vi "新建模板1.vi"() -> ()   [LabVIEW 2015]
uses:
  <vilib>/vision/NI_Vision_Development_Module.lvlib
  <vilib>/vision/driver/NI_Vision_Acquisition_Software.lvlib
  <vilib>/userdefined/High Color/IMAQdx.ctl
  <vilib>/vision/driver/IMAQdx.llb/IMAQdx Acquisition Mode.ctl
  <vilib>/vision/driver/IMAQdx.llb/IMAQdx Buffer Number Mode.ctl
panel:
  in  "选项卡控件":enum32{"选项卡 1"}(tab)
  out "Image":T1(plugin-control)
  out "Extracted Image":T1(plugin-control)
  in  "Stop":bool
  in  "保存按钮":bool
  in  "布尔":bool
  # "自定义模板界面"
  # "原始图片"
  # "模板图片"
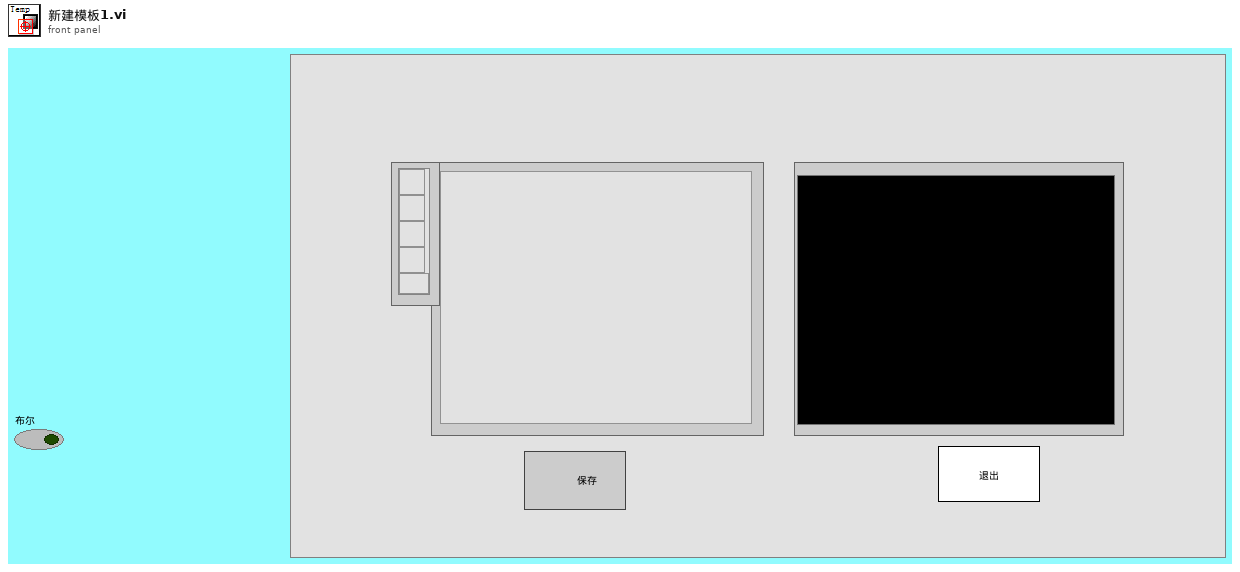
[diagram p1: front panel]
types:
  T1 = typedef "IMAQ Image.ctl" = refnum<image>
  T2 = cluster{"Zoom Tool":bool, "Selection Tool":bool, "Pan Tool":bool, "Point Tool":bool, "Line Tool":bool, "Rectangle Tool":bool, "Rotated Rectangle Tool":bool, "Polyline Tool":bool, "Polygon Tool":bool, "Freehand Tool":bool, "Closed Freehand Tool":bool, "Ellipse Tool":bool, "Annulus Tool":bool}
  T3 = typedef "NI_Vision_Acquisition_Software.lvlib/IMAQdx Buffer Number Mode.ctl" = enum32{"Next", "Last", "Buffer Number", "Every", "Last New"}
  T4 = typedef "NI_Vision_Acquisition_Software.lvlib/IMAQdx Acquisition Mode.ctl" = enum32{"One Shot", "Continuous"}
  T5 = typedef "IMAQdx.ctl" = refnum<k21>
  T6 = cluster{"Match Mode":u16, "Number of Matches Requested":i32, "Minimum Match Score":sgl, "SubPixel Accuracy":bool, "Rotation Angle Ranges":cluster{"Start":sgl, "End":sgl}[], "Show Search Area":bool, "Show Result":bool}
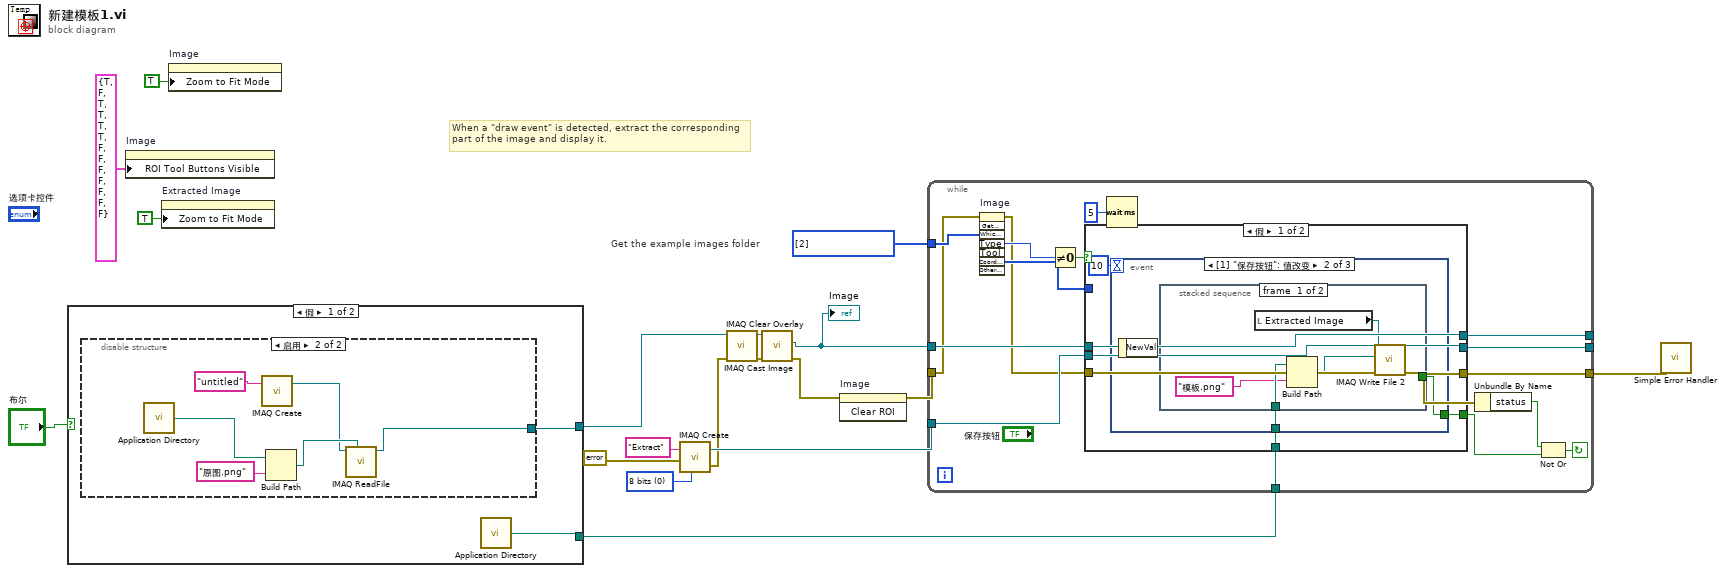
[diagram p0: block diagram]
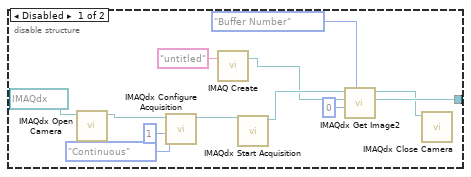
[diagram p2: hidden frame]
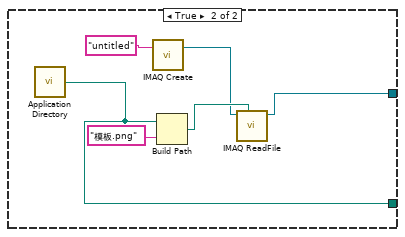
[diagram p3: hidden frame]
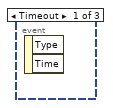
[diagram p4: hidden frame]
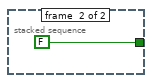
[diagram p5: hidden frame]
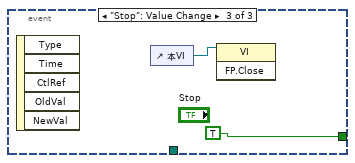
[diagram p6: hidden frame]
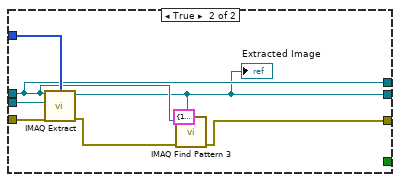
[diagram p7: hidden frame]
diagram:
  w14 = i32[] [2] items=["No  event", "Click event", "Draw event", "Move event", "Size event", "Scroll event", "Activate event", "Close event", "Double click event"] ("Events list (all)")
  w17 = u32 0 items=["8 bits", "16 bits", "Float", "Complex", "RGB", "HSL"] ("Image Type")
  # "When a \"draw event\" is detected, extract the corresponding part of the image and display it."
  # "Get the example images folder"
  n1 = case shown="假" "布尔" {
    tunnel: [w19 w39] -> w3
    tunnel: [w18 w38] -> w1
    frame False {
      n2 = disable-structure shown="启用" {
        disable-tunnel: [w21 w32] -> w19
        frame Disabled {
          n3 = call <vilib>:"IMAQdx Open Camera.vi"("Session In"=T5 "cam0") -> ("Session Out"=w30:T5)  [unwired: 9 in, 1 out]
          n4 = call <vilib>:"IMAQdx Configure Acquisition.vi"("Number of Buffers"=u32 1, "Continuous?"=IMAQdx_Acquisition_Mode."Continuous", "Session In"=w30) -> ("Session Out"=w27:T5)  [unwired: 7 in, 1 out]
          n5 = call "IMAQ Create"("Image Name"="untitled") -> ("New Image"=w24:T1)  [unwired: 4 in, 1 out]
          n6 = call <vilib>:"IMAQdx Start Acquisition.vi"("Session In"=w27) -> ("Session Out"=w26:T5)  [unwired: 9 in, 1 out]
          n7 = call <vilib>:"IMAQdx Get Image2.vi"("Buffer Number Mode (Next)"=IMAQdx_Buffer_Number_Mode."Buffer Number", "Buffer Number In"=u32 0, "Image In"=w24, "Session In"=w26) -> ("Image Out"=w21:T1, "Session Out"=w20:T5)  [unwired: 4 in, 2 out]
          n8 = call <vilib>:"IMAQdx Close Camera.vi"("Session In"=w20) -> ()  [unwired: 10 in, 1 out]
        }
        frame Enabled {
          n9 = call <vilib>:"Application Directory.vi"() -> ("Application Directory"=w33:path)
          n10 = call "IMAQ Create"("Image Name"="untitled") -> ("New Image"=w35:T1)  [unwired: 4 in, 1 out]
          n11 = Build Path(base path=w33, name or relative path="原图.png" ("名称或相对路径")) -> (appended path=w36:path)
          n12 = call "IMAQ ReadFile"("File Path"=w36, "Image"=w35) -> ("Image Out"=w32:T1)  [unwired: 5 in, 4 out]
        }
      }
      n13 = call <vilib>:"Application Directory.vi"() -> ("Application Directory"=w18:path)
    }
    frame True {
      n14 = call <vilib>:"Application Directory.vi"() -> ("Application Directory"=w38:path)
      n15 = call "IMAQ Create"("Image Name"="untitled") -> ("New Image"=w41:T1)  [unwired: 4 in, 1 out]
      n16 = Build Path(base path=w38, name or relative path="模板.png" ("名称或相对路径")) -> (appended path=w42:path)
      n17 = call "IMAQ ReadFile"("File Path"=w42, "Image"=w41) -> ("Image Out"=w39:T1)  [unwired: 5 in, 4 out]
    }
  }
  n18 = property on="Image" class="ImageControl"("ROI Tool Buttons Visible"=T2 {"Zoom Tool"=TRUE, "Selection Tool"=FALSE, "Pan Tool"=TRUE, "Point Tool"=TRUE, "Line Tool"=TRUE, "Rectangle Tool"=TRUE, "Rotated Rectangle Tool"=FALSE, "Polyline Tool"=FALSE, "Polygon Tool"=FALSE, "Freehand Tool"=FALSE, "Closed Freehand Tool"=FALSE, "Ellipse Tool"=FALSE, "Annulus Tool"=FALSE} ("ROI Tool Buttons Visible:All Elements")) -> ()  [unwired: 2 in, 2 out]
  n19 = property on="Extracted Image" class="ImageControl"("Zoom to Fit Mode"=TRUE) -> ()  [unwired: 2 in, 2 out]
  n20 = property on="Image" class="ImageControl"("Zoom to Fit Mode"=TRUE) -> ()  [unwired: 2 in, 2 out]
  n21 = call "IMAQ Create"("Image Name"="Extract", "Image Type"=w17, "error in (no error)"=errorcluster {"status"=FALSE, "code"=0, "source"=""}) -> ("New Image"=w15:T1, "error out"=w7:errorcluster)  [unwired: 1 in, 1 out]
  n22 = call "IMAQ Clear Overlay"("Image"=w3) -> ("Image Out"=w4:T1)  [unwired: 9 in, 1 out]
  n23 = call "IMAQ Cast Image"("error in (no error)"=w7, "Image Src"=w4) -> ("error out"=w8:errorcluster, "Image Dst Out"=w10:T1)  [unwired: 8 in]
  "Image" <- w10
  n24 = invoke on="Image" class="ImageControl" method="Clear ROI"(error in=w8) -> (error out=w13:errorcluster)  [unwired: 2 in, 2 out]
  n25 = while {
    tunnel: w15 -> [w54]
    tunnel: w10 -> [w56]
    tunnel: w13 -> [w46]
    tunnel: w14 -> [w55]
    tunnel: [w53] -> _
    tunnel: [w52] -> _
    tunnel: [w51] -> w5
    tunnel: w1 -> [w44]
    stop <- w49 continue-if-true
    n26 = invoke on="Image" class="ImageControl" method="Get Last Event"(error in=w46, "Which Events"=w55) -> (error out=w45:errorcluster, "Type"=w57:i32, "Coordinates"=w58:i32[])  [unwired: 6 in, 5 out]
    n27 = Not Equal To 0?(x=w57) -> (x != 0?=w59:bool)
    n28 = case shown="假" w59 {
      tunnel: w58 -> [_ w82]
      tunnel: w45 -> [w63 w81]
      tunnel: w56 -> [w65 w78]
      tunnel: [w63 w76] -> w51
      tunnel: [w64 w75] -> w52
      tunnel: w54 -> [w64 w80]
      tunnel: [w65 w78] -> w53
      tunnel: [w62 _] -> w47
      tunnel: w44 -> [w60 _]
      frame False {
        n29 = event shown="[1] \"保存按钮\": 值改变" {
          selector: _ -> [_ _ _]
          dyn-events: _ -> [_ _ _]
          timeout: 10 -> [_ _ _]
          tunnel: [_ w67 TRUE] -> w62
          tunnel: w60 -> [_ w66 _]
          event Timeout {
            n30 = event-data() -> ()  [unwired: 1 in, 2 out]
          }
          event "保存按钮": Value Change {
            n31 = event-data() -> ()  [unwired: 1 in, 1 out]
            n32 = stacked-sequence {
              tunnel: [_ FALSE] -> w67
              tunnel: w66 -> [w70 _]
              frame #0 {
                n33 = local read "Extracted Image"() -> (w71:T1)
                n34 = Build Path(base path=w70, name or relative path="模板.png" ("字符串")) -> (appended path=w69:path)
                n35 = call-poly "IMAQ Write File 2"("File Path"=w69, "Image"=w71) -> ()  [unwired: 8 in, 2 out]
              }
              frame #1 {
              }
            }
          }
          event "Stop": Value Change {
            n36 = event-data() -> ()  [unwired: 1 in, 5 out]
            n37 = control-ref of="本VI"() -> (w73:refnum<vi>)
            n38 = invoke class="VI" method="FP.Close"(reference=w73) -> ()  [unwired: 2 in, 3 out]
          }
        }
      }
      frame True {
        n39 = call "IMAQ Extract"("Optional Rectangle"=w82, "error in (no error)"=w81, "Image Dst"=w80, "Image Src"=w78) -> ("error out"=w79:errorcluster, "Image Dst Out"=w75:T1)  [unwired: 2 in, 4 out]
        "Extracted Image" <- w75
        n40 = call "IMAQ Find Pattern 3"("Settings"=T6 {"Match Mode"=1, "Number of Matches Requested"=1, "Minimum Match Score"=500.0, "SubPixel Accuracy"=TRUE, "Rotation Angle Ranges"=[{"Start"=-180.0, "End"=180.0}], "Show Search Area"=FALSE, "Show Result"=TRUE}, "Template"=w75, "error in (no error)"=w79, "Image"=w78) -> ("error out"=w76:errorcluster)  [unwired: 2 in, 5 out]
      }
    }
    n41 = Wait (ms)(milliseconds to wait=u32 5) -> ()  [unwired: 1 out]
    n42 = Unbundle By Name(w51) -> ("status"=w50:bool)
    n43 = Not Or(1:w47, 2:w50) -> (0:w49:bool)
  }
  n44 = call <vilib>:"Simple Error Handler.vi"("error in (no error)"=w5) -> ()  [unwired: 1 in, 8 out]
